vi "PS_Scope.vi"(10 "Label":string, 11 "Waveforms":waveform(dbl)[](array[waveform])) -> (3 "PS Waveform":cluster{"f0":dbl, "df":dbl, "magnitude":dbl[]}(graph))   [LabVIEW 2019, in "DSP.lvclass"]
uses:
  DSP.lvclass
  <vilib>/measure/maspectr.llb/FFT Power Spectrum and PSD for 1 Chan.vi
  <vilib>/measure/NI_MAPro.lvlib
panel:
  in  "index":i32
  in  "restart avg":bool
  out "done?":bool
  out "averages":dbl=10.0
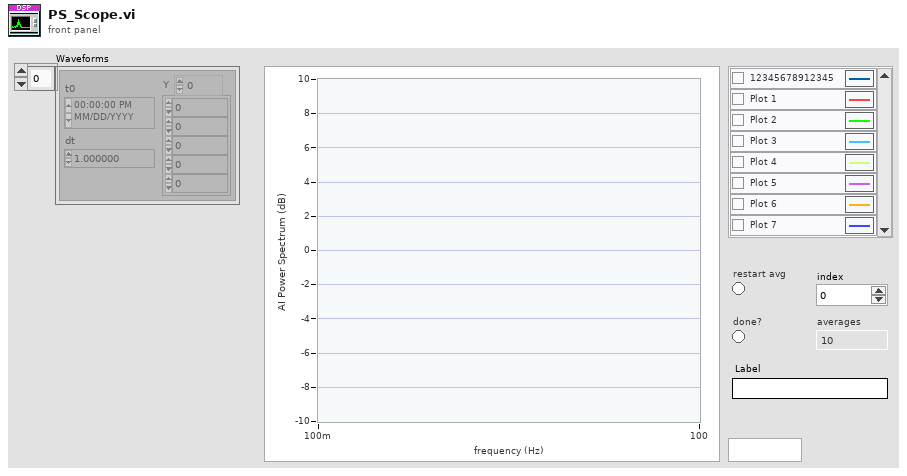
[diagram p1: front panel]
types:
  T1 = enum16{"No averaging", "Vector averaging", "RMS averaging", "Peak hold"}
  T2 = cluster{"averaging mode":enum16{"No averaging", "Vector averaging", "RMS averaging", "Peak hold"}, "weighting mode":enum16{"Linear", "Exponential"}, "number of averages":u32}
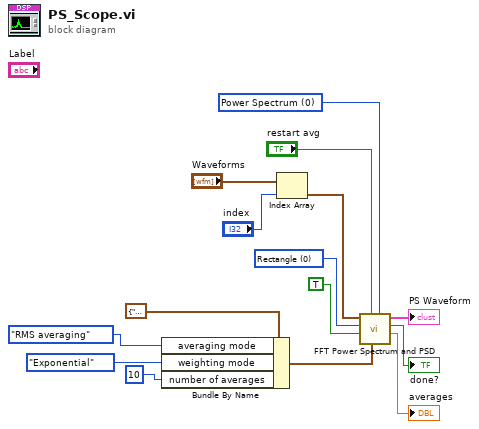
[diagram p0: block diagram]
diagram:
  w10 = u16 0 items=["Rectangle", "Hanning"] ("window")
  w14 = u16 0 items=["Power Spectrum", "Power Spectral Density"] ("export mode")
  n1 = Bundle By Name(cluster=T2 {"averaging mode"=enum."No averaging", "weighting mode"=enum."Exponential", "number of averages"=10} ("averaging parameters"), "averaging mode"=T1."RMS averaging", "weighting mode"=enum16{"Linear", "Exponential"}."Exponential", "number of averages"=u32 10 ("# averages")) -> (w8:T2)
  n2 = Index Array(array="Waveforms", index="index") -> (element=w2:waveform(dbl))
  n3 = call-poly <vilib>:"FFT Power Spectrum and PSD.vi"("export mode"=w14, "averaging parameters"=w8, "restart averaging (F)"="restart avg", "dB On (F)"=TRUE, "window"=w10, "time signal"=w2) -> ("averages completed"=→"averages":dbl, "averaging done"=→"done?":bool, "Power Spectrum / PSD"=→"PS Waveform":cluster{"f0":dbl, "df":dbl, "magnitude":dbl[]})  [unwired: 2 in, 1 out]
